vi "TCP Close.vi"(8 "Error In":errorcluster, 11 "LINX Decice Config":T1) -> (0 "Error Out":errorcluster, 3 "LINX Decice Config":T1)   [LabVIEW 2014, in "LMH-LINX.lvlib" / "Device.lvlib"]
uses:
  <vilib>/MakerHub/LINX/Private/Device/Device.lvlib
  <vilib>/MakerHub/LINX/Private/Device/Type Defs/LINX Device Config.ctl
  <vilib>/MakerHub/LINX/Private/Type Defs/Interface.ctl
  <vilib>/MakerHub/LINX/Private/Device/Type Defs/TCP Config.ctl
  <vilib>/MakerHub/LINX/Private/Device/Type Defs/Channels.ctl
  <vilib>/MakerHub/LINX/LMH-LINX.lvlib
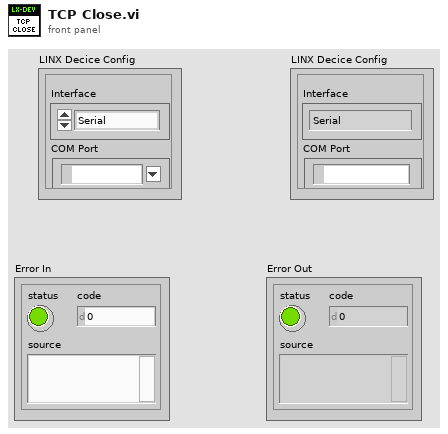
[diagram p1: front panel]
types:
  T1 = typedef "LMH-LINX.lvlib/Device.lvlib/LINX Device Config.ctl" = cluster{"Interface":T2, "COM Port":refnum<visa-resource-name>, "TCP Configuration":T3, "Device Family":u8, "Device ID":u8, "Device Name":string, "TCP Ref":refnum<k5>, "Channels":T4}
  T2 = typedef "LMH-LINX.lvlib/Interface.ctl" = enum16{"Serial", "TCP"}
  T3 = typedef "LMH-LINX.lvlib/Device.lvlib/TCP Config.ctl" = cluster{"IP Address":string, "Port":u16}
  T4 = typedef "LMH-LINX.lvlib/Channels.ctl" = cluster{"DI":u8[], "DO":u8[], "AI":u8[], "AO":u8[], "PWM":u8[], "QE":u8[], "UART":u8[], "I2C 2":u8[], "SPI":u8[], "CAN":u8[], "Servo":u8[], "AI Ref (V)":dbl, "AI Resolution (Bits)":u8, "AO Ref (V)":dbl, "AO Resolution (Bits)":u8}
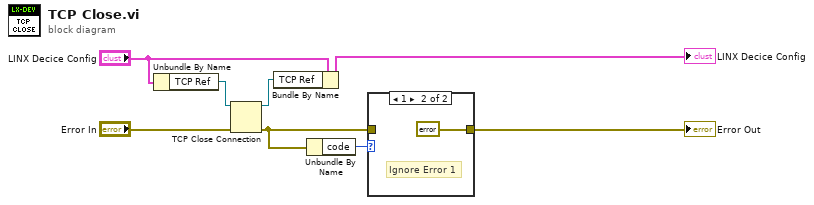
[diagram p0: block diagram]
diagram:
  n1 = Unbundle By Name("LINX Decice Config") -> ("TCP Ref"=w8:refnum<k5>)
  n2 = TCP Close Connection(connection ID=w8, error in (no error)="Error In") -> (connection ID out=w6:refnum<k5>, error out=w1:errorcluster)  [unwired: 1 in]
  n3 = Bundle By Name(cluster="LINX Decice Config", "TCP Ref"=w6) -> (→"LINX Decice Config":T1)
  n4 = Unbundle By Name(w1) -> ("code"=w3:i32)
  n5 = case shown="1" w3 {
    tunnel: [w9 errorcluster {"status"=FALSE, "code"=0, "source"=""} ("error out")] -> w2
    tunnel: w1 -> [w9 _]
    frame 0, Default {
    }
    frame 1 {
      # "Ignore Error 1"
    }
  }
  "Error Out" <- w2
